vi "Execute Bookmark Action.vi"(8 "Error In":errorcluster, 9 "Tree Tag":string, 10 "Menu Tag":string, 11 "Bookmarks":T1[](array[typedef])) -> (0 "Error Out":errorcluster)   [LabVIEW 2018, in "Bookmark Manager.lvlib"]
uses:
  Bookmark Manager.lvlib
  Controls/BMark_Bookmark Data.ctl
  Controls/BMark_VI_Identifier.ctl
  <vilib>/addons/analyzer/_analyzerctrls.llb/VIAnCtl Analysis App Info.ctl
  Toolkit/Toolkit.lvlib
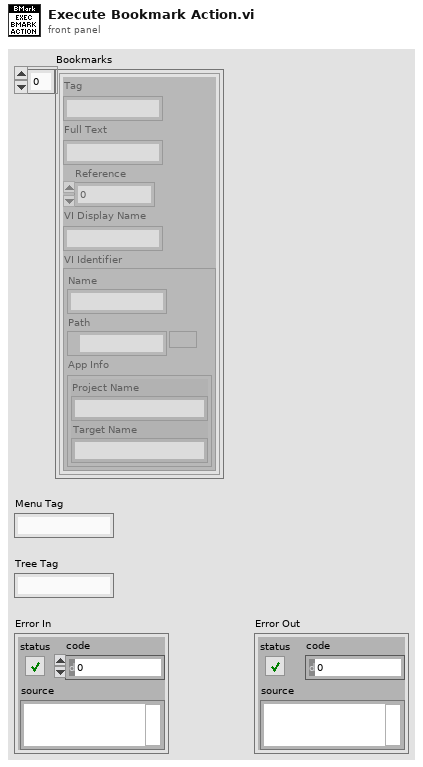
[diagram p1: front panel]
types:
  T1 = typedef "Bookmark Manager.lvlib/BMark_Bookmark Data.ctl" = cluster{"Tag":string, "Full Text":string, "Reference":i32, "VI Display Name":string, "VI Identifier":T2}
  T2 = typedef "Bookmark Manager.lvlib/BMark_VI_Identifier.ctl" = cluster{"Name":string, "Path":path, "App Info":T3}
  T3 = typedef "VIAnCtl Analysis App Info.ctl" = cluster{"Project Name":string, "Target Name":string}
  T4 = enum32{"Bad", "Idle", "Run top level", "Running"}
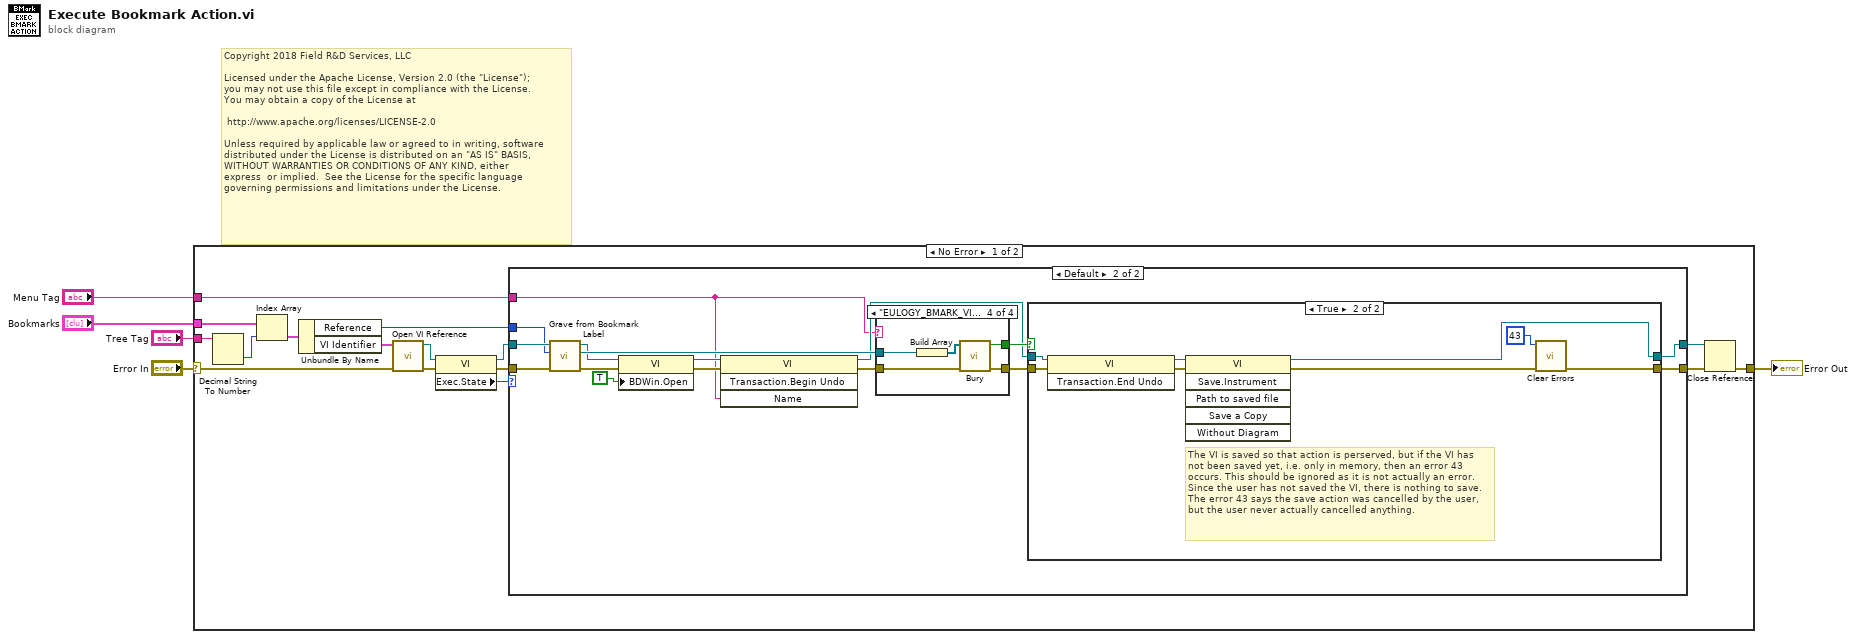
[diagram p0: block diagram]
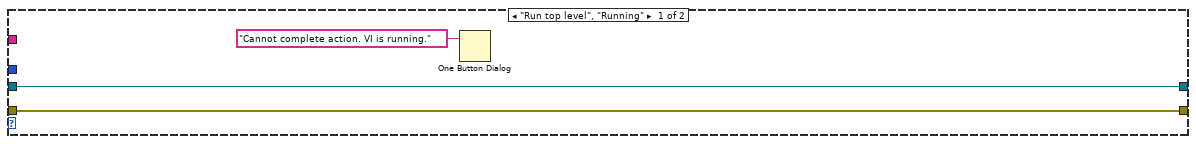
[diagram p2: hidden frame]
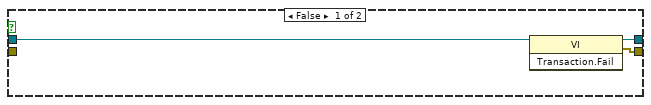
[diagram p3: hidden frame]
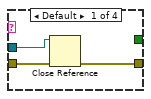
[diagram p4: hidden frame]
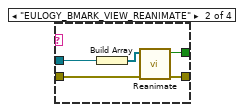
[diagram p5: hidden frame]
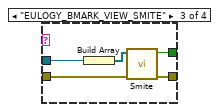
[diagram p6: hidden frame]
diagram:
  # "Copyright 2018 Field R&D Services, LLC\n\nLicensed under the Apache License, Version 2.0 (the \"License\");\nyou may not use this file except in compliance with the License.\nYou may obtain a copy of the License at\n\n\thttp://www.apache.org/licenses/LICENSE-2.0\n\nUnless required by applicable law or agreed to in writing, software\ndistributed under the License is distributed on an \"AS IS\" BASIS,\nWITHOUT WARRANTIES OR CONDITIONS OF ANY KIND, either \nexpress  or implied.  See the License for the specific language \ngoverning permissions and limitations under the License."
  n1 = case shown="No Error" "Error In" {
    selector: "Error In" -> [w19 w70]
    tunnel: "Tree Tag" -> [w18 _]
    tunnel: "Bookmarks" -> [w17 _]
    tunnel: [w21 w70] -> w4
    tunnel: "Menu Tag" -> [w20 _]
    frame No Error {
      n2 = Decimal String To Number(string=w18) -> (number=w16:i32)  [unwired: 2 in, 1 out]
      n3 = Index Array(array=w17, index=w16) -> (element=w10:T1)
      n4 = Unbundle By Name(w10) -> ("Reference"=w9:i32, "VI Identifier"=w6:T2)
      n5 = call "Open VI Reference.vi"("Error In"=w19, "VI Identifier"=w6) -> ("Error Out"=w8:errorcluster, "VI"=w7:refnum<vi>)  [unwired: 8 in]
      n6 = property class="VI"(reference=w7, error in=w8) -> (reference out=w13:refnum<vi>, error out=w14:errorcluster, "Exec.State"=w15:T4)
      n7 = case shown="Default" w15 {
        tunnel: [w23 w30] -> w11
        tunnel: w14 -> [w23 w40]
        tunnel: w13 -> [w24 w38]
        tunnel: [w24 w31] -> w12
        tunnel: w20 -> [_ w25]
        tunnel: w9 -> [_ w36]
        frame "Run top level", "Running" {
          n8 = One Button Dialog(message="Cannot complete action. VI is running.") -> ()  [unwired: 1 in, 1 out]
        }
        frame Default {
          n9 = call "Grave from Bookmark Label.vi"("Error In"=w40, "Bookmark ID"=w36, "VI In"=w38) -> ("Error Out"=w34:errorcluster, "Grave"=w39:refnum<vi>, "VI Out"=w37:refnum<vi>)  [unwired: 6 in]
          n10 = property class="VI"(reference=w37, error in=w34, "BDWin.Open"=TRUE ("Block Diagram Window:Open")) -> (reference out=w35:refnum<vi>, error out=w33:errorcluster)
          n11 = invoke class="VI" method="Transaction.Begin Undo"(reference=w35, error in=w33, "Name"=w25) -> (reference out=w27:refnum<vi>, error out=w26:errorcluster)  [unwired: 1 in, 2 out]
          n12 = case shown="\"EULOGY_BMARK_VIEW_BURY\"" w25 {
            tunnel: w39 -> [w54 w59 w64 w69]
            tunnel: [w52 w57 w61 w67] -> w29
            tunnel: [_ w56 w60 w66] -> w28
            tunnel: w26 -> [w53 w55 w62 w65]
            frame Default {
              n13 = Close Reference(reference=w54, error in (no error)=w53) -> (error out=w52:errorcluster)
            }
            frame "EULOGY_BMARK_VIEW_REANIMATE" {
              n14 = Build Array(w59) -> (w58:refnum<vi>[])
              n15 = call "Reanimate.vi"("Error In"=w55, "Graves"=w58) -> ("Error Out"=w57:errorcluster, "Change Made?"=w56:bool)  [unwired: 8 in]
            }
            frame "EULOGY_BMARK_VIEW_SMITE" {
              n16 = Build Array(w64) -> (w63:refnum<vi>[])
              n17 = call "Smite.vi"("Error In"=w62, "Graves"=w63) -> ("Error Out"=w61:errorcluster, "Change Made?"=w60:bool)  [unwired: 8 in]
            }
            frame "EULOGY_BMARK_VIEW_BURY" {
              n18 = Build Array(w69) -> (w68:refnum<vi>[])
              n19 = call "Bury.vi"("Error In"=w65, "Graves"=w68) -> ("Error Out"=w67:errorcluster, "Change Made?"=w66:bool)  [unwired: 8 in]
            }
          }
          n20 = case shown="True" w28 {
            tunnel: [w43 w50] -> w31
            tunnel: [w42 w45] -> w30
            tunnel: w29 -> [_ w47]
            tunnel: w27 -> [w41 w46]
            frame False {
              n21 = invoke class="VI" method="Transaction.Fail"(reference=w41) -> (reference out=w43:refnum<vi>, error out=w42:errorcluster)  [unwired: 2 in, 1 out]
            }
            frame True {
              # "The VI is saved so that action is perserved, but if the VI has not been saved yet, i.e. only in memory, then an error 43 occurs. This should be ignored as it is not actually an error. Since the user has not saved the VI, there is nothing to save. The error 43 says the save action was cancelled by the user, but the user never actually cancelled anything."
              n22 = invoke class="VI" method="Transaction.End Undo"(reference=w46, error in=w47) -> (reference out=w51:refnum<vi>, error out=w49:errorcluster)  [unwired: 1 in, 1 out]
              n23 = invoke class="VI" method="Save.Instrument"(reference=w51, error in=w49) -> (reference out=w50:refnum<vi>, error out=w48:errorcluster)  [unwired: 4 in, 4 out]
              n24 = call <vilib>:"Clear Errors.vi"("error in (no error)"=w48, "specific error code to clear (0: all)"=43) -> ("error out"=w45:errorcluster)  [unwired: 4 in, 1 out]
            }
          }
        }
      }
      n25 = Close Reference(reference=w12, error in (no error)=w11) -> (error out=w21:errorcluster)
    }
    frame Error {
    }
  }
  "Error Out" <- w4
